vi "DumpBanks.vi"(10 "Experiment State":T1={"Send Trigger 3"=FALSE, "error"={"status"=FALSE, "code"=0, "source"=""}, "Tasks"={"Fiber15 MP Task"="MyVoltageTask", "Read Slow AI"="", "Fiber Bank DIO"="", "Fiber7 MP Task"="MyVoltageTask", "TaskArray"=[]}, "Channels"={"6133 Channels"=[], "Trigger Source"="", "Edge Type"=10280, "Samples Per Channel"=[], "#Pre-Trigger Samples"=[], "Sample Rate 2.5Ms/s Max"=[]}, "Dev 10 DIO"="", "Dev5"="", "Fiber Triggers 2"=[{"Delay (s)"=2.559999942779541, "Pulse width (s)"=0.009999999776482582, "Active"=TRUE, "Channel Name"="Fiber 8", "counter"="PXI1Slot8/ctr7"}], "MP7"=FALSE, "MP15"=FALSE, "PXI Slot 2"={"PXI Slot 2 Handle"="PXI1Slot2", "source terminal"="GlobalSoftwareTrigger"}, "# of Control DIOs"=0, "Bank DIO Settings"=[], "Purge Duration (s)"=5, "Interlock Override"=FALSE, "Current Raw Voltages, Slot &"=[], "Bank Control"={"Bank Enables"={"Gun1 Enable"=FALSE, "Gun2 Enable"=FALSE, "InnerSol Enable"=FALSE, "OuterSol1 Enable"=FALSE, "Outer2 Enable"=FALSE, "Gun3 Enable"=FALSE}, "Voltages"={"Gun1 Voltage"=0.0, "Gun2 Voltage"=0.0, "Gun3 Voltage"=0.0, "InnerSol Voltage"=0.0, "OuterSol1 Voltage"=0.0, "OuterSol2 Voltage"=0.0}, "Set Points"={"Gun1 Setpoint"=0.0, "Gun2 Setpoint"=0.0, "Gun3 Setpoint"=0.0, "InnerSol Setpoint"=0.0, "OuterSol1 Setpoint"=0.0, "OuterSol2 Setpoint"=0.0}}, "Waveform Data"=[], "Next Shot#"="0", "Slot 7, Last Shot Scaled Voltages"=[], "Data Run Description"="", "Next Shot Data"=["599", "6/18/2009", "4:08PM", "Ziemba", "Bank Testing", "-7.142518", "-8.256295", "-6.893030", "-5.120022", "-0.001235", "-0.001559", "-0.000910", "-0.001235", "-0.001235", "-0.001235", "-0.001235", "0.114909", "-0.000586", "-0.000586", "0.684598", "1.197512"], "Headers"=[], "Html Shot Log View"=FALSE, "ShotLog Headers"=path "", "ShotLog Data"=path "", "Enable Bank Control"=FALSE, "6602  Slot8"={"Slot 8 Trigger Source"="", "Slot 8 Clock Source"="", "Trigger Channel Tasks"=[]}, "6602  Slot 9"={"Slot 9 Clock Source"="", "Slot 9 Trigger Source"="", "Trigger Channel Tasks"=[]}, "Total Sample Time (us)"=[], "Pre-Trigger Time (us)"=[], "Fiber Triggers"=[{"Delay (s)"=2.559999942779541, "Pulse width (s)"=0.009999999776482582, "Active"=TRUE, "Channel Name"="ns", "counter"=""}], "System Message"=""} {"Fiber Triggers"."Pulse width (s)" format="%.3p"; "Fiber Triggers"."Delay (s)" format="%.3p"; "Pre-Trigger Time (us)" format="%#_6f"; "Total Sample Time (us)" format="%#_6f"; "Current Raw Voltages, Slot &" format="%0.2f"; "Fiber Triggers 2"."Pulse width (s)" format="%.3p"; "Fiber Triggers 2"."Delay (s)" format="%.3p"; "Channels"."Sample Rate 2.5Ms/s Max" format="%#_3p"; "Channels"."Edge Type" items=["Rising"=10280, "Falling"=10171]}) -> (2 "Experiment State":T1={"Send Trigger 3"=FALSE, "error"={"status"=FALSE, "code"=0, "source"=""}, "Tasks"={"Fiber15 MP Task"="MyVoltageTask", "Read Slow AI"="", "Fiber Bank DIO"="", "Fiber7 MP Task"="MyVoltageTask", "TaskArray"=[]}, "Channels"={"6133 Channels"=[], "Trigger Source"="", "Edge Type"=10280, "Samples Per Channel"=[], "#Pre-Trigger Samples"=[], "Sample Rate 2.5Ms/s Max"=[]}, "Dev 10 DIO"="", "Dev5"="", "Fiber Triggers 2"=[{"Delay (s)"=2.559999942779541, "Pulse width (s)"=0.009999999776482582, "Active"=TRUE, "Channel Name"="Fiber 8", "counter"="PXI1Slot8/ctr7"}], "MP7"=FALSE, "MP15"=FALSE, "PXI Slot 2"={"PXI Slot 2 Handle"="PXI1Slot2", "source terminal"="GlobalSoftwareTrigger"}, "# of Control DIOs"=0, "Bank DIO Settings"=[], "Purge Duration (s)"=5, "Interlock Override"=FALSE, "Current Raw Voltages, Slot &"=[], "Bank Control"={"Bank Enables"={"Gun1 Enable"=FALSE, "Gun2 Enable"=FALSE, "InnerSol Enable"=FALSE, "OuterSol1 Enable"=FALSE, "Outer2 Enable"=FALSE, "Gun3 Enable"=FALSE}, "Voltages"={"Gun1 Voltage"=0.0, "Gun2 Voltage"=0.0, "Gun3 Voltage"=0.0, "InnerSol Voltage"=0.0, "OuterSol1 Voltage"=0.0, "OuterSol2 Voltage"=0.0}, "Set Points"={"Gun1 Setpoint"=0.0, "Gun2 Setpoint"=0.0, "Gun3 Setpoint"=0.0, "InnerSol Setpoint"=0.0, "OuterSol1 Setpoint"=0.0, "OuterSol2 Setpoint"=0.0}}, "Waveform Data"=[], "Next Shot#"="0", "Slot 7, Last Shot Scaled Voltages"=[], "Data Run Description"="", "Next Shot Data"=["599", "6/18/2009", "4:08PM", "Ziemba", "Bank Testing", "-7.142518", "-8.256295", "-6.893030", "-5.120022", "-0.001235", "-0.001559", "-0.000910", "-0.001235", "-0.001235", "-0.001235", "-0.001235", "0.114909", "-0.000586", "-0.000586", "0.684598", "1.197512"], "Headers"=[], "Html Shot Log View"=FALSE, "ShotLog Headers"=path "", "ShotLog Data"=path "", "Enable Bank Control"=FALSE, "6602  Slot8"={"Slot 8 Trigger Source"="", "Slot 8 Clock Source"="", "Trigger Channel Tasks"=[]}, "6602  Slot 9"={"Slot 9 Clock Source"="", "Slot 9 Trigger Source"="", "Trigger Channel Tasks"=[]}, "Total Sample Time (us)"=[], "Pre-Trigger Time (us)"=[], "Fiber Triggers"=[{"Delay (s)"=2.559999942779541, "Pulse width (s)"=0.009999999776482582, "Active"=TRUE, "Channel Name"="ns", "counter"=""}], "System Message"=""} {"Fiber Triggers"."Pulse width (s)" format="%.3p"; "Fiber Triggers"."Delay (s)" format="%.3p"; "Pre-Trigger Time (us)" format="%#_6f"; "Total Sample Time (us)" format="%#_6f"; "Current Raw Voltages, Slot &" format="%0.2f"; "Fiber Triggers 2"."Pulse width (s)" format="%.3p"; "Fiber Triggers 2"."Delay (s)" format="%.3p"; "Channels"."Sample Rate 2.5Ms/s Max" format="%#_3p"; "Channels"."Edge Type" items=["Rising"=10280, "Falling"=10171]})   [LabVIEW 2013]
uses:
  Controls/ExperimentStateCluster.ctl
  <vilib>/DAQmx/write.llb/DAQmx Write (Digital 1D Bool NChan 1Samp 1Line).vi
  <vilib>/DAQmx/miscellaneous.llb/DAQmx Fill In Error Info.vi
types:
  T1 = typedef "ExperimentStateCluster.ctl" = cluster{"Send Trigger 3":bool, "error":errorcluster, "Tasks":cluster{"Fiber15 MP Task":refnum<k21>, "Read Slow AI":refnum<k21>, "Fiber Bank DIO":refnum<k21>, "Fiber7 MP Task":refnum<k21>, "TaskArray":refnum<k21>[]}, "Channels":cluster{"6133 Channels":tag[], "Trigger Source":tag, "Edge Type":i32, "Samples Per Channel":i32[], "#Pre-Trigger Samples":u32[], "Sample Rate 2.5Ms/s Max":dbl[]}, "Dev 10 DIO":refnum<k21>, "Dev5":refnum<k21>, "Fiber Triggers 2":cluster{"Delay (s)":dbl, "Pulse width (s)":dbl, "Active":bool, "Channel Name":string, "counter":tag}[], "MP7":bool, "MP15":bool, "PXI Slot 2":cluster{"PXI Slot 2 Handle":refnum<k15>, "source terminal":string}, "# of Control DIOs":i32, "Bank DIO Settings":bool[], "Purge Duration (s)":u32, "Interlock Override":bool, "Current Raw Voltages, Slot &":dbl[], "Bank Control":cluster{"Bank Enables":cluster{"Gun1 Enable":bool, "Gun2 Enable":bool, "InnerSol Enable":bool, "OuterSol1 Enable":bool, "Outer2 Enable":bool, "Gun3 Enable":bool}, "Voltages":cluster{"Gun1 Voltage":dbl, "Gun2 Voltage":dbl, "Gun3 Voltage":dbl, "InnerSol Voltage":dbl, "OuterSol1 Voltage":dbl, "OuterSol2 Voltage":dbl}, "Set Points":cluster{"Gun1 Setpoint":dbl, "Gun2 Setpoint":dbl, "Gun3 Setpoint":dbl, "InnerSol Setpoint":dbl, "OuterSol1 Setpoint":dbl, "OuterSol2 Setpoint":dbl}}, "Waveform Data":waveform(dbl)[][], "Next Shot#":string, "Slot 7, Last Shot Scaled Voltages":string[], "Data Run Description":string, "Next Shot Data":string[], "Headers":string[], "Html Shot Log View":bool, "ShotLog Headers":path, "ShotLog Data":path, "Enable Bank Control":bool, "6602  Slot8":cluster{"Slot 8 Trigger Source":tag, "Slot 8 Clock Source":tag, "Trigger Channel Tasks":refnum<k21>[]}, "6602  Slot 9":cluster{"Slot 9 Clock Source":tag, "Slot 9 Trigger Source":tag, "Trigger Channel Tasks":refnum<k21>[]}, "Total Sample Time (us)":dbl[], "Pre-Trigger Time (us)":dbl[], "Fiber Triggers":cluster{"Delay (s)":dbl, "Pulse width (s)":dbl, "Active":bool, "Channel Name":string, "counter":tag}[], "System Message":string}
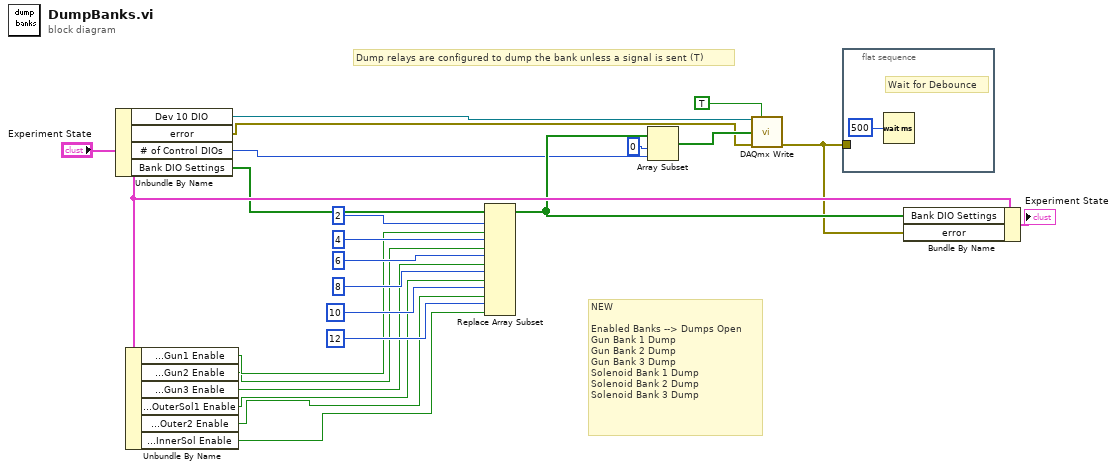
[diagram p0: block diagram]
diagram:
  # "Dump relays are configured to dump the bank unless a signal is sent (T)"
  # "NEW\n\nEnabled Banks --> Dumps Open\nGun Bank 1 Dump\nGun Bank 2 Dump\nGun Bank 3 Dump\nSolenoid Bank 1 Dump\nSolenoid Bank 2 Dump\nSolenoid Bank 3 Dump"
  n1 = Unbundle By Name("Experiment State") -> ("Dev 10 DIO"=w23:refnum<k21>, "error"=w8:errorcluster, "# of Control DIOs"=w9:i32, "Bank DIO Settings"=w19:bool[])
  n2 = Unbundle By Name("Experiment State") -> ("Bank Control.Bank Enables.Gun1 Enable"=w6:bool, "Bank Control.Bank Enables.Gun2 Enable"=w5:bool, "Bank Control.Bank Enables.Gun3 Enable"=w4:bool, "Bank Control.Bank Enables.OuterSol1 Enable"=w3:bool, "Bank Control.Bank Enables.Outer2 Enable"=w2:bool, "Bank Control.Bank Enables.InnerSol Enable"=w1:bool)
  n3 = Replace Array Subset(array=w19, new element #1=w6, index #1=2 ("index"), new element #2=w5, index #2=4 ("index"), new element #3=w4, index #3=6 ("index"), new element #4=w3, index #4=8 ("index"), new element #5=w2, index #5=10 ("index"), new element #6=w1, index #6=12 ("index")) -> (w20:bool[])
  n4 = Array Subset(array=w20, index=0, length=w9) -> (w16:bool[])
  n5 = call-poly <vilib>:"DAQmx Write.vi"("task/channels in"=w23, "auto start"=TRUE, "data"=w16, "error in"=w8) -> ("error out"=w7:errorcluster)  [unwired: 11 out]
  n6 = flat-sequence {
    tunnel: w7 -> [_]
    frame #0 {
      # "Wait for Debounce"
      n7 = Wait (ms)(milliseconds to wait=u32 500) -> ()  [unwired: 1 out]
    }
  }
  n8 = Bundle By Name(cluster="Experiment State", "Bank DIO Settings"=w20, "error"=w7) -> (→"Experiment State":T1)
